vi "Get Paths to Icon Editor Files in LV Installation.vi"() -> (2 "relative paths":path[](array[path]), 3 "absolute paths":path[](array[path]))   [LabVIEW 2020]
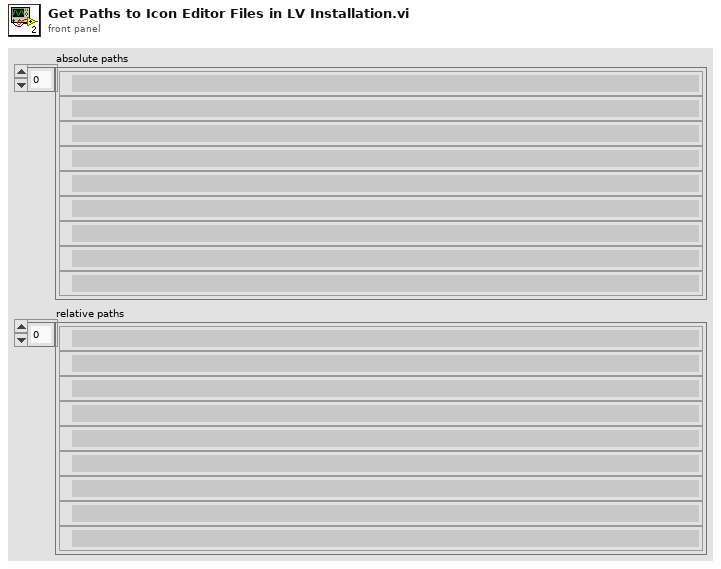
[diagram p1: front panel]
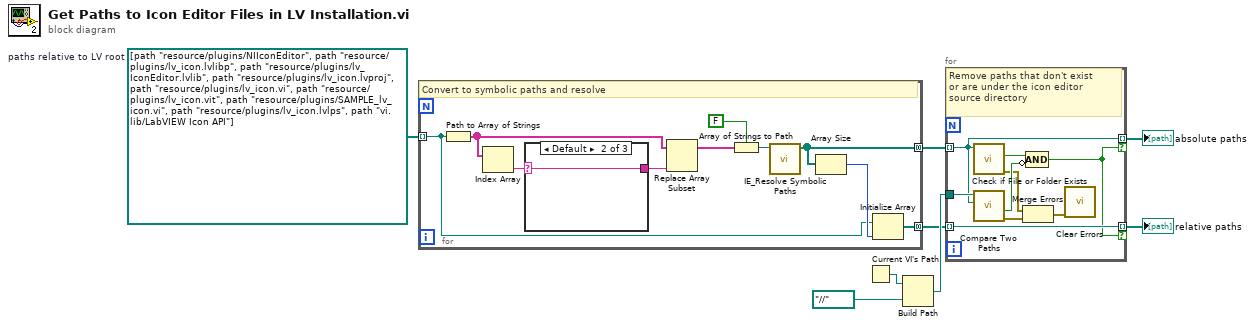
[diagram p0: block diagram]
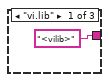
[diagram p2: hidden frame]
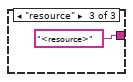
[diagram p3: hidden frame]
diagram:
  w8 = path[] [path "resource/plugins/NIIconEditor", path "resource/plugins/lv_icon.lvlibp", path "resource/plugins/lv_IconEditor.lvlib", path "resource/plugins/lv_icon.lvproj", path "resource/plugins/lv_icon.vi", path "resource/plugins/lv_icon.vit", path "resource/plugins/SAMPLE_lv_icon.vi", path "resource/plugins/lv_icon.lvlps", path "vi.lib/LabVIEW Icon API"]  # paths relative to LV root
  n1 = for {
    tunnel: w8 -> [w11] mode=indexing
    tunnel: [w10] -> w2 mode=concatenating
    tunnel: [w9] -> w4 mode=concatenating
    # "Convert to symbolic paths and resolve"
    n2 = Path to Array of Strings(0:w11) -> (2:w17:string[])  [unwired: 1 out]
    n3 = Index Array(array=w17) -> (element=w18:string)  [unwired: 1 in]
    n4 = case shown="Default" w18 {
      selector: w18 -> [_ w20 _]
      tunnel: ["<vilib>" w20 "<resource>"] -> w16
      frame "vi.lib" {
      }
      frame Default {
      }
      frame "resource" {
      }
    }
    n5 = Replace Array Subset(array=w17, new element=w16) -> (w15:string[])  [unwired: 1 in]
    n6 = Array of Strings to Path(0:w15, 1:FALSE ("relative")) -> (2:w13:path)
    n7 = call <resource>:"IE_Resolve Symbolic Paths.vi"("symbolic path"=w13) -> ("resolved paths"=w9:path[])  [unwired: 10 in]
    n8 = Array Size(array=w9) -> (size(s)=w12:i32)
    n9 = Initialize Array(w11, w12) -> (w10:path[])
  }
  n10 = Current VI's Path() -> (path=w7:path)
  n11 = Build Path(base path=w7, name or relative path=path "../../..") -> (appended path=w5:path)
  n12 = for {
    tunnel: w5 -> [w30]
    tunnel: w4 -> [w28] mode=indexing
    tunnel: [w29] -> w3 mode=indexing if=w25
    tunnel: w2 -> [w29] mode=indexing
    tunnel: [w28] -> w1 mode=indexing if=w25
    # "Remove paths that don't exist\nor are under the icon editor\nsource directory"
    n13 = call <vilib>:"Check if File or Folder Exists.vi"("path"=w28) -> ("error out"=w24:errorcluster, "file or folder exists?"=w26:bool)  [unwired: 8 in, 1 out]
    n14 = call <vilib>:"Compare Two Paths.vi"("Path 2"=w28, "Path 1"=w30) -> ("error out"=w23:errorcluster, "Path 2 Relative to Path 1?"=w27:bool)  [unwired: 6 in, 2 out]
    n15 = Merge Errors(w24, w23) -> (w22:errorcluster)
    n16 = Compound Arithmetic op=AND(w26, invert w27) -> (w25:bool)
    n17 = call <vilib>:"Clear Errors.vi"("error in (no error)"=w22) -> ()  [unwired: 5 in, 2 out]
  }
  "absolute paths" <- w1
  "relative paths" <- w3
